vi "Auton Extension Control.vi"(6 "Setpoint":dbl, 11 "Feedback":dbl) -> (2 "PWM 7 Output":dbl)   [LabVIEW 2011]
uses:
  Robot Global Data.vi
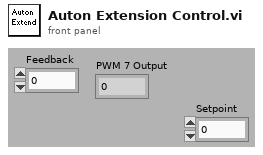
[diagram p1: front panel]
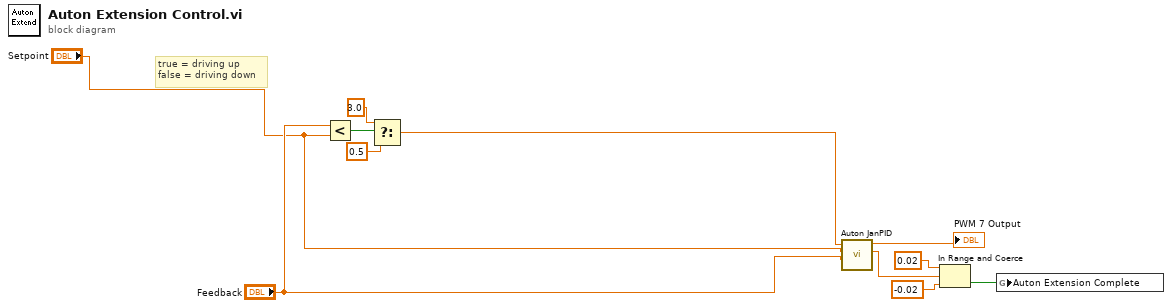
[diagram p0: block diagram]
diagram:
  # "true = driving up\nfalse = driving down"
  n1 = Less?(x="Feedback", y="Setpoint") -> (x < y?=w8:bool)
  n2 = Select(t=3.0, s=w8, f=0.5) -> (s? t:f=w5:dbl)
  n3 = call "Auton JanPID.vi"("Feedback"="Feedback", "Setpoint"="Setpoint", "P"=w5) -> ("Error"=w2:dbl, "Motor Output"=→"PWM 7 Output":dbl)  [unwired: 1 in, 6 out]
  n4 = In Range and Coerce(upper limit=0.02, x=w2, lower limit=-0.02) -> (In Range?=w9:bool)  [unwired: 1 out]
  n5 = global write "Robot Global Data.vi" "Auton Extension Complete"(w9) -> ()
